vi "FlatToRichResponse.vi"(5 "OutputClusterType":T1, 11 "InputCluster":T2) -> (3 "OutputCluster":T1)   [LabVIEW 2019, in "Generated_server.lvlib"]
uses:
  Generated_server.lvlib
  Response_Flat.ctl
  Response.ctl
  Response_response_oneof/Response_response_oneof.lvclass
  Response_response_oneof/Response_response_oneof.lvclass/Response_response_oneof.ctl
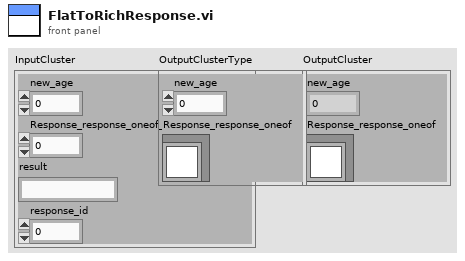
[diagram p1: front panel]
types:
  T1 = typedef "Generated_server.lvlib/Response.ctl" = cluster{"new_age":i32, "Response_response_oneof":refnum<class "Response_response_oneof.lvclass">}
  T2 = typedef "Generated_server.lvlib/Response_Flat.ctl" = cluster{"new_age":i32, "Response_response_oneof_selected_index":i32, "result":string, "response_id":i32}
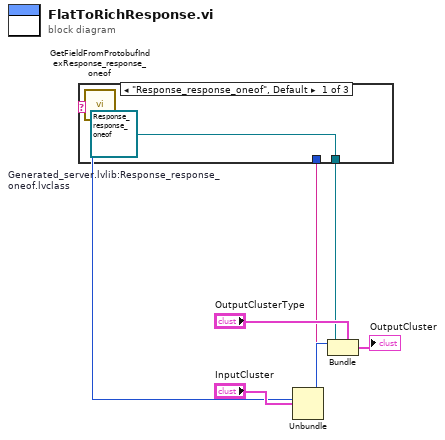
[diagram p0: block diagram]
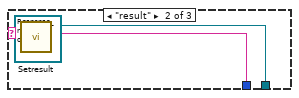
[diagram p2: hidden frame]
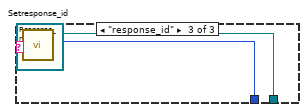
[diagram p3: hidden frame]
diagram:
  n1 = Unbundle "Unbundle"("InputCluster") -> ("new_age"=w6:i32, "Response_response_oneof_selected_index"=w5:i32, "result"=w2:string, "response_id"=w1:i32)
  n2 = call "GetFieldFromProtobufIndexResponse_response_oneof.vi"("protobuf index"=w5) -> ("oneof field name"=w4:string)
  n3 = case "Response_response_oneof" shown="\"Response_response_oneof\", Default" w4 {
    tunnel: [w10 w12 w15] -> w3
    tunnel: w2 -> [_ w13 _]
    tunnel: w1 -> [_ _ w16]
    frame "Response_response_oneof", Default {
      w10 = refnum<class "Response_response_oneof.lvclass"> refnum  # Generated_server.lvlib:Response_response_oneof.lvclass
    }
    frame "result" {
      n4 = call "Setresult.vi"("Set_Val"=w13, "OneOfTemplate in"=refnum<class "Response_response_oneof.lvclass"> refnum) -> ("OneOfTemplate out"=w12:refnum<class "Response_response_oneof.lvclass">)  [unwired: 8 in, 1 out]
    }
    frame "response_id" {
      n5 = call "Setresponse_id.vi"("Set_Val"=w16, "OneOfTemplate in"=refnum<class "Response_response_oneof.lvclass"> refnum) -> ("OneOfTemplate out"=w15:refnum<class "Response_response_oneof.lvclass">)  [unwired: 8 in, 1 out]
    }
  }
  n6 = Bundle "Bundle"(cluster="OutputClusterType", "new_age"=w6, "Response_response_oneof"=w3) -> (→"OutputCluster":T1)
